vi "WriteActor.vi"(7 "ConcreteActor":refnum<class "ConcreteActor.lvclass">, 11 "Actor":refnum<class "Actor.lvclass">) -> (5 "ConcreteActor":refnum<class "ConcreteActor.lvclass">)   [LabVIEW 2020, in "_Template.lvlib" / "ActorTemplate.lvlib" / "{{Name}}.lvlib" / "ConcreteActor.lvclass"]
uses:
  ConcreteActor.lvclass
  jettl/jettl/Actor/Actor.lvclass
  ConcreteActor.lvclass/ConcreteActor.ctl
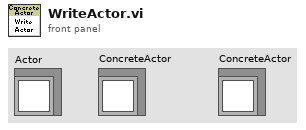
[diagram p1: front panel]
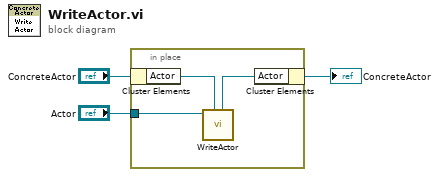
[diagram p0: block diagram]
diagram:
  n1 = in-place {
    in-place-border: "Actor" -> [w4]
    n2 = in-place-cluster #1("ConcreteActor") -> ("Actor"=w6:refnum<class "Actor.lvclass">)
    n3 = call-dynamic "WriteActor.vi"(7:"Actor"=w6, 11:"Actor"=w4) -> ("Actor"=w5:refnum<class "Actor.lvclass">)  [unwired: 9 in]
    n4 = in-place-cluster #1("Actor"=w5) -> (→"ConcreteActor":refnum<class "ConcreteActor.lvclass">)
  }
